vi "Text control 1 v0.1.vi"() -> ()   [LabVIEW 2016]
panel:
  in  "Panel Controls 2":T1={"Emergency Stop"=refnum, "TransGraph Max"=1e-05, "Text/Graph (text=false)"=TRUE, "TransGraph Min"=1e-11} {"TransGraph Min" format="%.2e"; "TransGraph Max" format="%.2e"}
  out "Currently running:":string="#output s 0 0 0 -0.008 0.008 0.002"
  in  "Lines left to run:":string
  in  "Standby":T2
  in  "Full Reset":bool
  in  "SMU4":cluster{"on/off":bool, "Voltage":dbl} {"Voltage" min=-100.0 max=100.0 format="%.2f"}
  in  "Source/Drain\nRange":u8(slide)=6 max=11 scale=0.0..11.0
  in  "Source/Drain\nRange mode":u16(ring) items=["Auto", "Limited", "Fixed"]
  in  "Gate Range":u8(slide)=6 max=11 scale=0.0..11.0
  in  "Gate Range\nmode":u16(ring) items=["Auto", "Limited", "Fixed"]
  in  "Gate":T3={"Gate Start"=0.0, "Gate Stop"=2.0, "Gate Step (linear only)"=1.0, "Gate Compliance"=0.0001, "Gate PComp"=0.0, "Range mode"=0, "Range"=6} {"Range" max=11 scale=0.0..11.0; "Range mode" items=["Auto", "Limited", "Fixed"]; "Gate PComp" format="%^.2e"; "Gate Compliance" format="%^.2e"; "Gate Step (linear only)" format="%^.4e"; "Gate Stop" format="%^.4e"; "Gate Start" format="%^.4e"}
  in  "Drain 2":T4={"Drain Start"=0.0, "Drain Stop"=2.0, "Drain Compliance"=0.0001, "Drain Step"=1.0, "Drain PComp"=0.0, "Range mode"=0, "Range"=6} {"Range" max=11 scale=0.0..11.0; "Range mode" items=["Auto", "Limited", "Fixed"]; "Drain PComp" format="%^.2e"; "Drain Step" format="%^.4e"; "Drain Compliance" format="%^.2e"; "Drain Stop" format="%^.4e"; "Drain Start" format="%^.4e"}
  in  "Timings 2":T5={"integration time"=0, "Short/Long integration time"=0.00064, "hold time (sec)"=0.0, "delay time (sec)"=0.0, "Step Time (0 disables)"=0.0, "sweep method"=0, "Pulse period"=0.005, "Base voltage"=0.0, "Pulse width"=0.0005} {"Pulse width" min=0.0005 max=0.1 step=0.0001 format="%.4f"; "Base voltage" format="%^.4e"; "Pulse period" min=0.005 max=1.0 step=0.0001 format="%.4f"; "sweep method" items=["Continuous", "Pulsed"]; "Step Time (0 disables)" format="%.2f"; "delay time (sec)" format="%.4f"; "hold time (sec)" format="%.4f"; "Short/Long integration time" format="%^.0e"; "integration time" scale=0.0..2.0}
  in  "Panel Controls":T6={"Emergency Stop"=refnum, "TransGraph Max"=1e-05, "Text/Graph (text=false)"=TRUE} {"TransGraph Max" format="%.2e"}
  in  "Interrupt run":bool
  in  "Drain: Compliance":dbl=0.001 format="%.8f"
  in  "Gate: Compliance":dbl=0.001 format="%.8f"
  out "Path":path=path "C:/users/rlp38/09Apr2009LTtesting/test2.txt"
  in  "hold time /s":dbl format="%.2f"
  in  "delay time /s":dbl format="%.2f"
  in  "integration time":u32(slide)=1 max=2 step=1 scale=0.0..2.0
  in  "Integration time (short)":dbl=0.0019 min=8e-05 max=0.0019 step=8e-05 format="%^.0e"
  in  "Integration time (long)":dbl=0.32 min=0.04 max=2.0 step=0.02 format="%.2f"
  in  "Step delay /s":dbl format="%.2f"
  in  "Program":string="#pulsedstressV d 0.03 20 0 0.5 0.0827 5\n#\n#itime m\n#gaterangemode a\n#drainrangemode a\n#pulsed on 0.05 0 0.02\n#transfer d -10 40 1 5 40 35\n#transfer d -10 40 1 5 40 35\n#transfer d -10 40 1 5 40 35\n#output d 0 40 20 0 40 1\n#\n#\n#sample 1 0.008 221 6 0.003\n#samplei 400e-6 200 6 0.002 0.1\n#vsu2pulse -10 4\n#\n#stressV 0.016 0.03 2e-4 0.1e-3 11\n#stressI 220e-7 0.08 15\n#transfer s -1 1 0.5 -0.005 0.005 0.005\n#output s 0 0 0 -0.008 0.008 0.002\n"
  # "Syntax:\nitime [s|m|l]\ngaterangemode [a|l|f]\ndrainrangemode [a|l|f]\npulsed [on|off] PulsePeriod(sec) PulseBaseVoltage PulseONWidth(sec)\nstandby [on l off]\nwait NumMilliseconds\nwait-min NumMinutes\n# texthere = comment\ntransfer [s|d] VgStart VgStop VgStep VdStart VdStop VdStep\noutput [s|d] VgStart VgStop VgStep VdStart VdStop VdStep\nsample Vg Vd NumSamples Time(s) SampleInterval(s)\nsamplei Idg NumSamples Time(s) SampleInterval(s) VDGcompliance\n# if in doubt use SampleInterval(s) = 0.004\nstressV VG VD IGcompliance IDcompliance Duration(sec)\nstressI IDG VDGcompliance Duration(sec)\nvsu2pulse Bias Duration(s)\npulsedstressV [s|d] VEstop VgON VgOFF Period(s) PulseONwidth(s) Vd\nsample-fpp Vg Vd NumSamples Time\nresample-fpp Vg Vd\ntransfer-fpp [s|d] VgStart VgStop VgStep VdStart VdStop VdStep\noutput-fpp [s|d] VgStart VgStop VgStep VdStart VdStop VdStep"
  # "100 samples is approx 13s with medium integration"
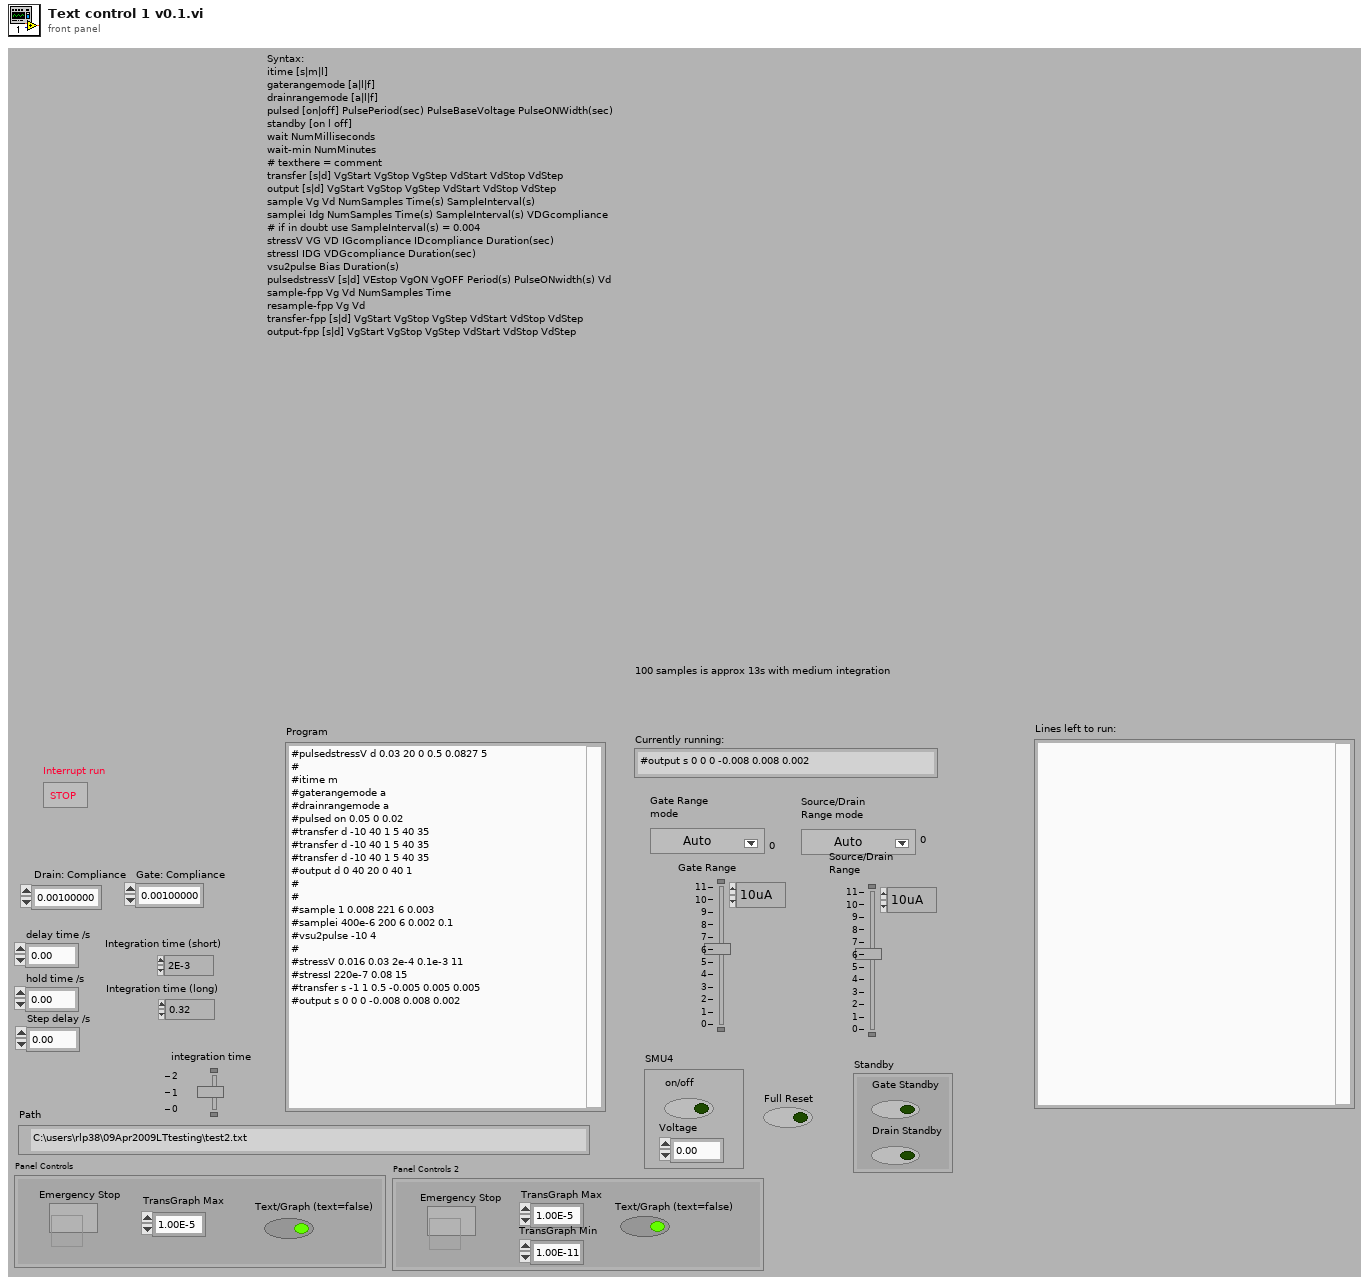
[diagram p1: front panel]
types:
  T1 = cluster{"Emergency Stop":refnum<vi>, "TransGraph Max":dbl, "Text/Graph (text=false)":bool, "TransGraph Min":dbl}
  T2 = cluster{"Gate Standby":bool, "Drain Standby":bool}
  T3 = cluster{"Gate Start":dbl, "Gate Stop":dbl, "Gate Step (linear only)":dbl, "Gate Compliance":dbl, "Gate PComp":dbl, "Range mode":u16, "Range":u8}
  T4 = cluster{"Drain Start":dbl, "Drain Stop":dbl, "Drain Compliance":dbl, "Drain Step":dbl, "Drain PComp":dbl, "Range mode":u16, "Range":u8}
  T5 = cluster{"integration time":u32, "Short/Long integration time":dbl, "hold time (sec)":dbl, "delay time (sec)":dbl, "Step Time (0 disables)":dbl, "sweep method":u16, "Pulse period":dbl, "Base voltage":dbl, "Pulse width":dbl}
  T6 = cluster{"Emergency Stop":refnum<vi>, "TransGraph Max":dbl, "Text/Graph (text=false)":bool}
  T7 = enum16{"open", "replace", "create", "open or create", "replace or create", "replace or create with confirmation"}
  T8 = cluster{"V2 Start":dbl, "V2 Step":dbl, "Number of points":i32}
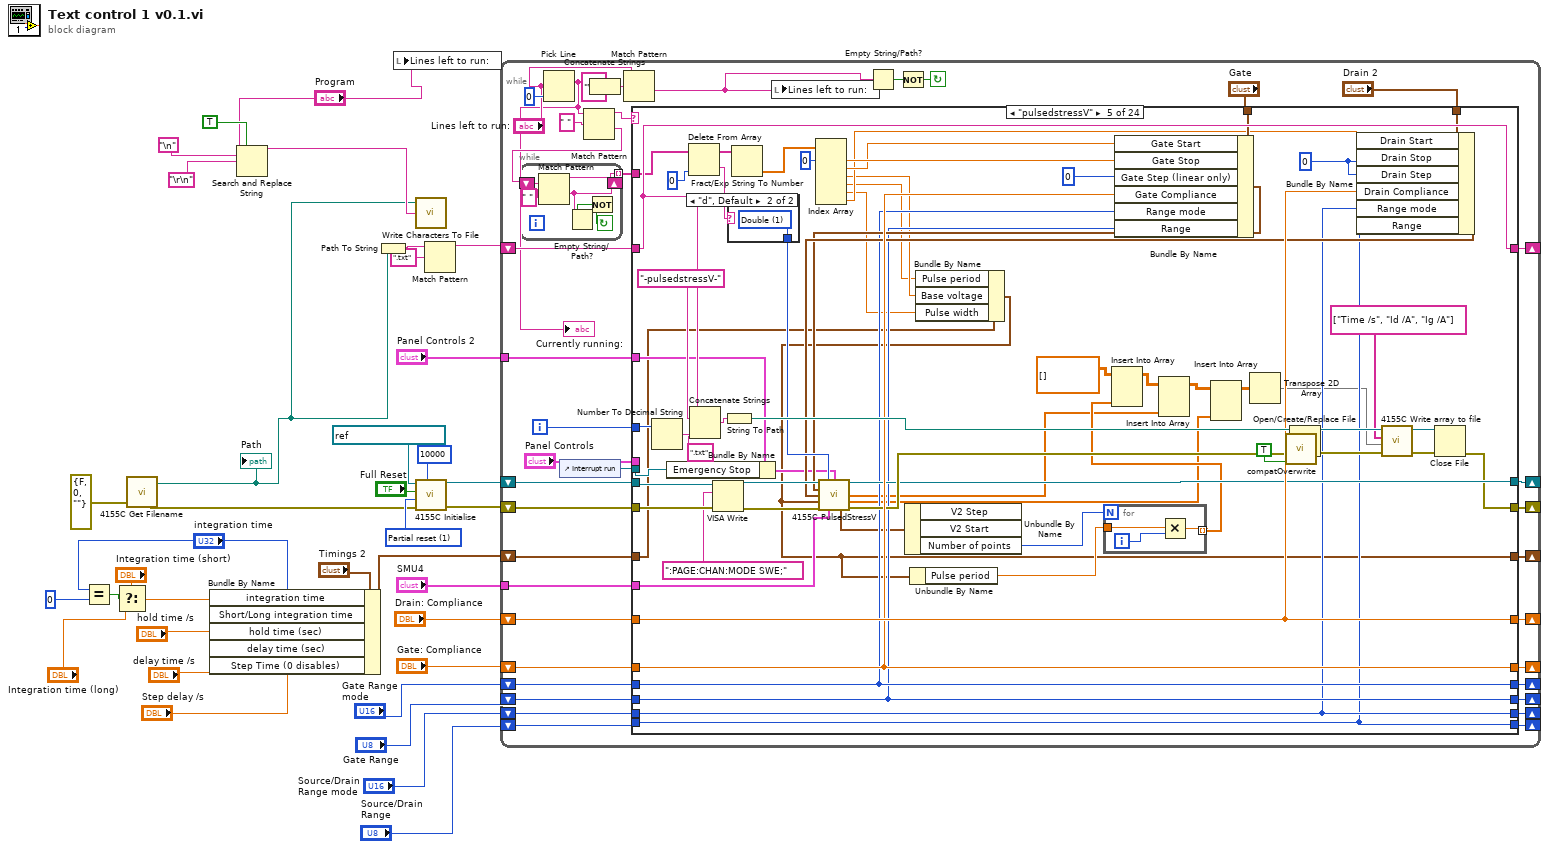
[diagram p0: block diagram]
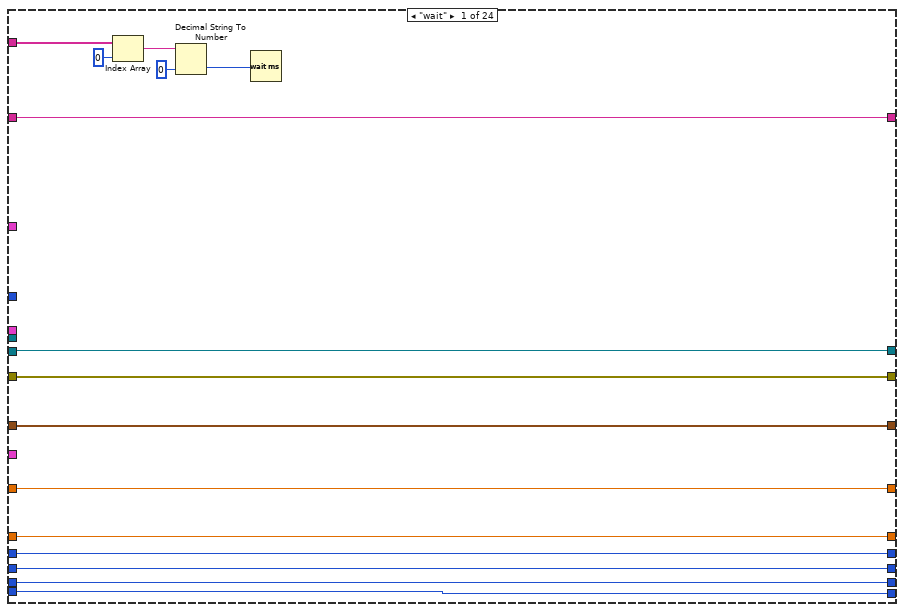
[diagram p2: hidden frame]
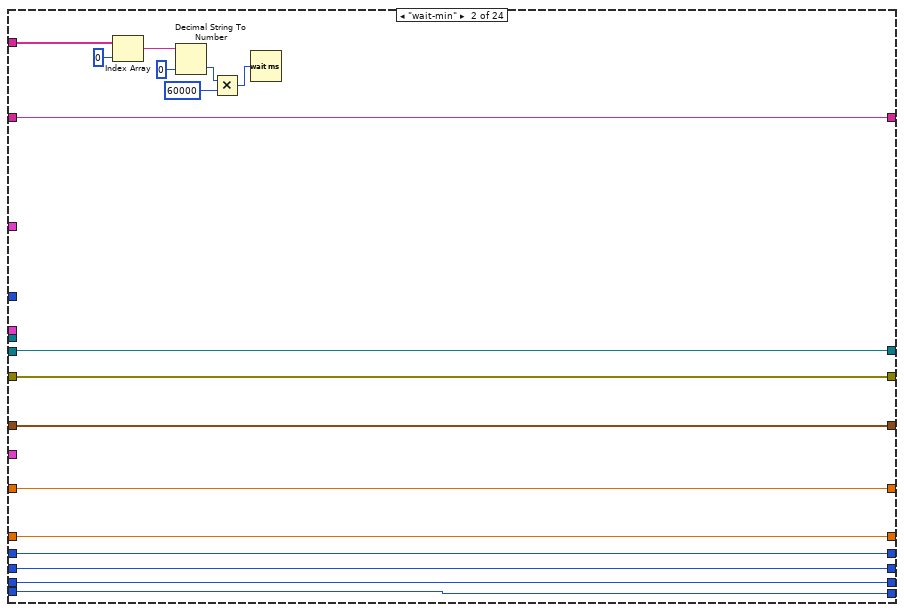
[diagram p3: hidden frame]
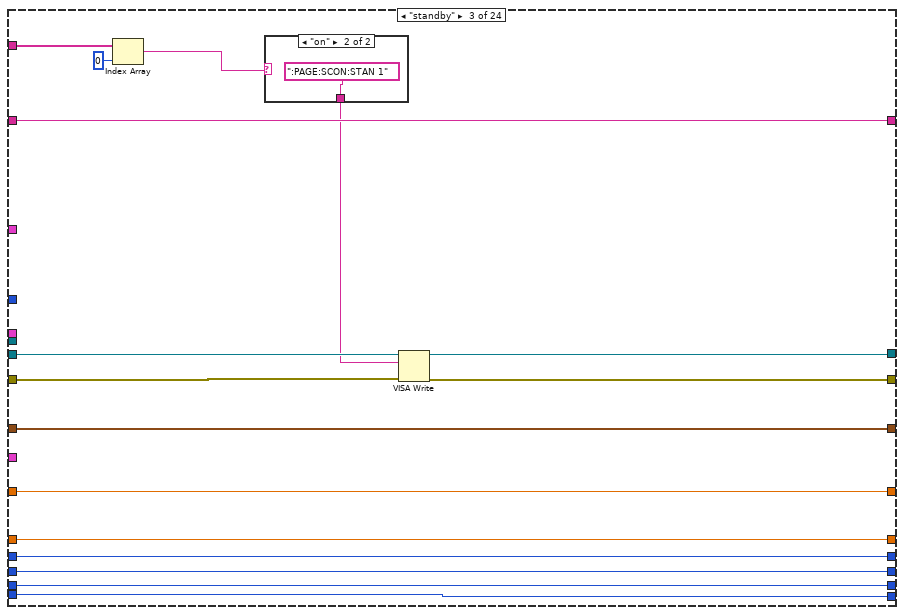
[diagram p4: hidden frame]
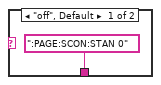
[diagram p5: hidden frame]
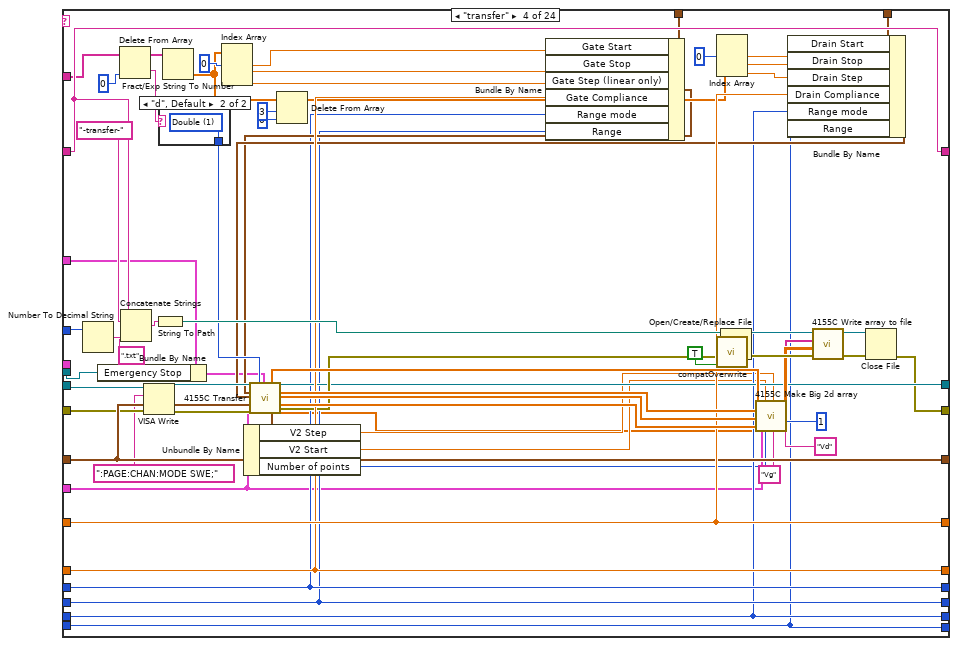
[diagram p6: hidden frame]
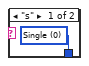
[diagram p7: hidden frame]
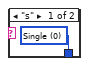
[diagram p8: hidden frame]
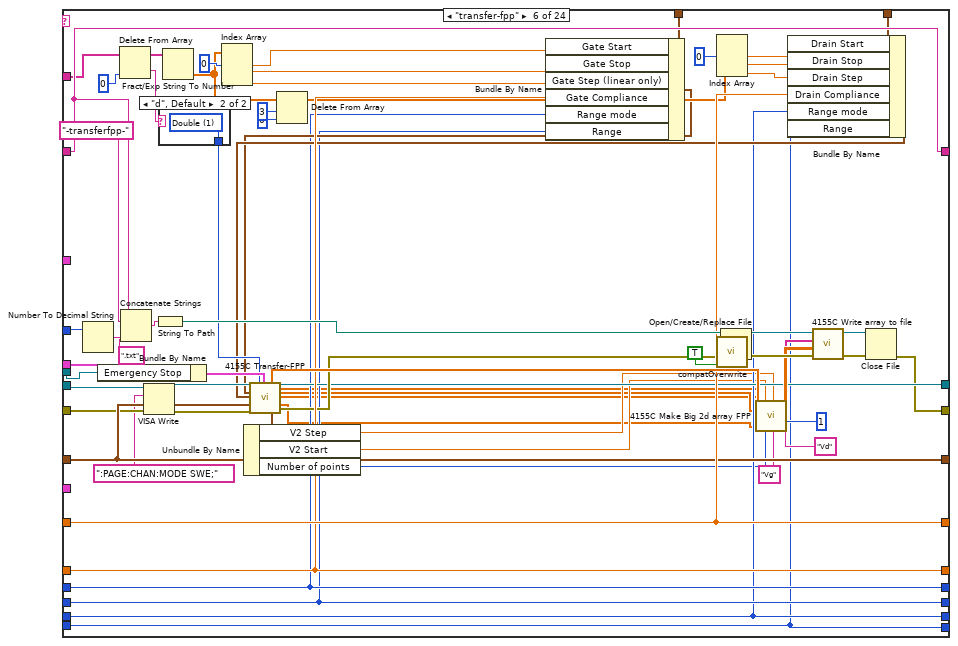
[diagram p9: hidden frame]
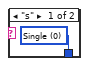
[diagram p10: hidden frame]
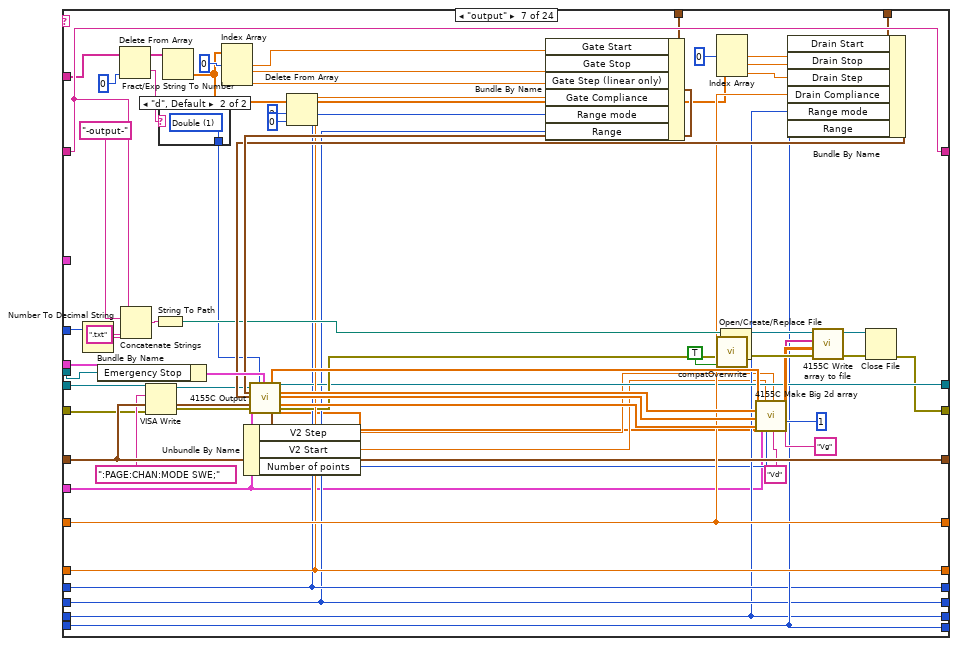
[diagram p11: hidden frame]
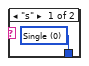
[diagram p12: hidden frame]
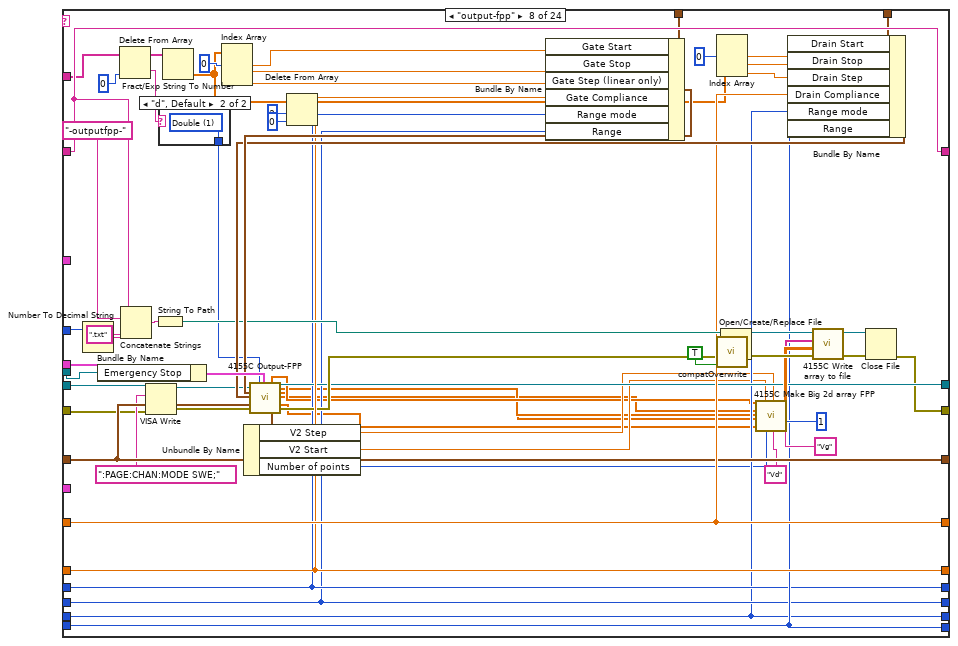
[diagram p13: hidden frame]
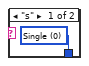
[diagram p14: hidden frame]
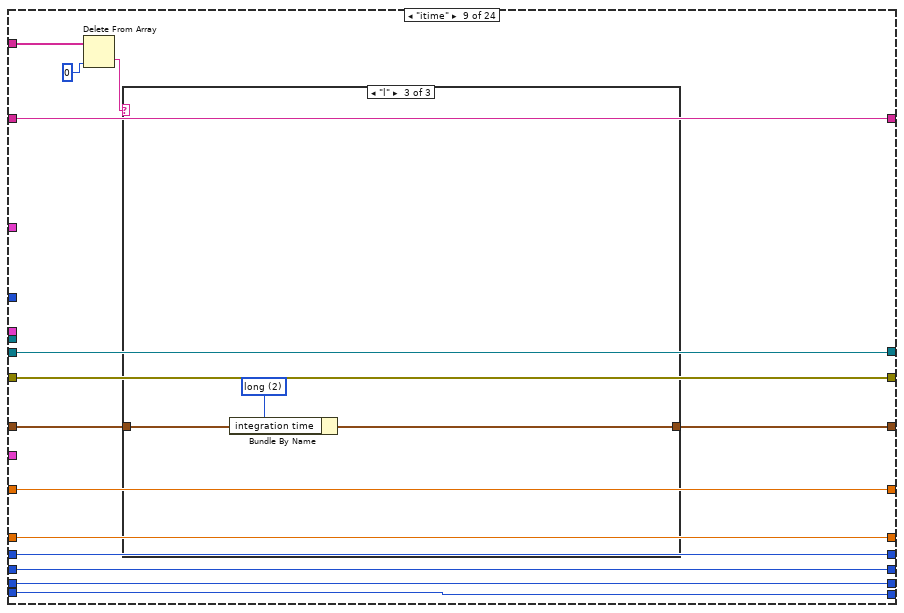
[diagram p15: hidden frame]
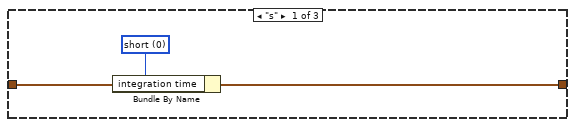
[diagram p16: hidden frame]
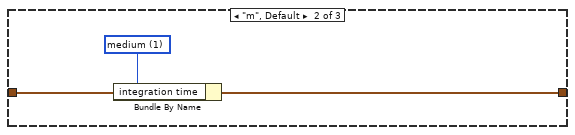
[diagram p17: hidden frame]
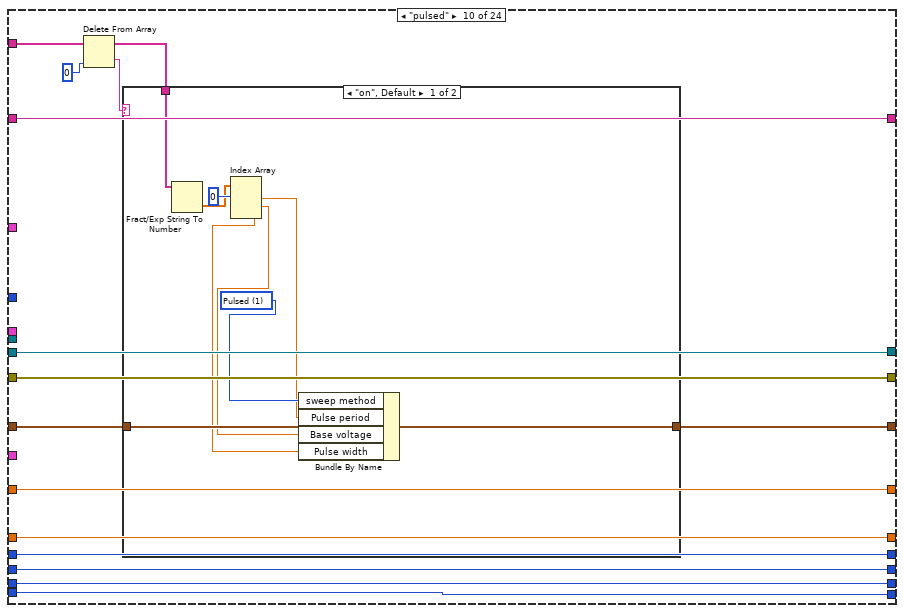
[diagram p18: hidden frame]
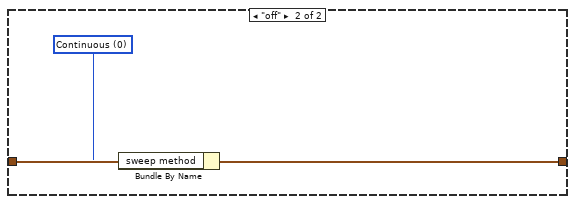
[diagram p19: hidden frame]
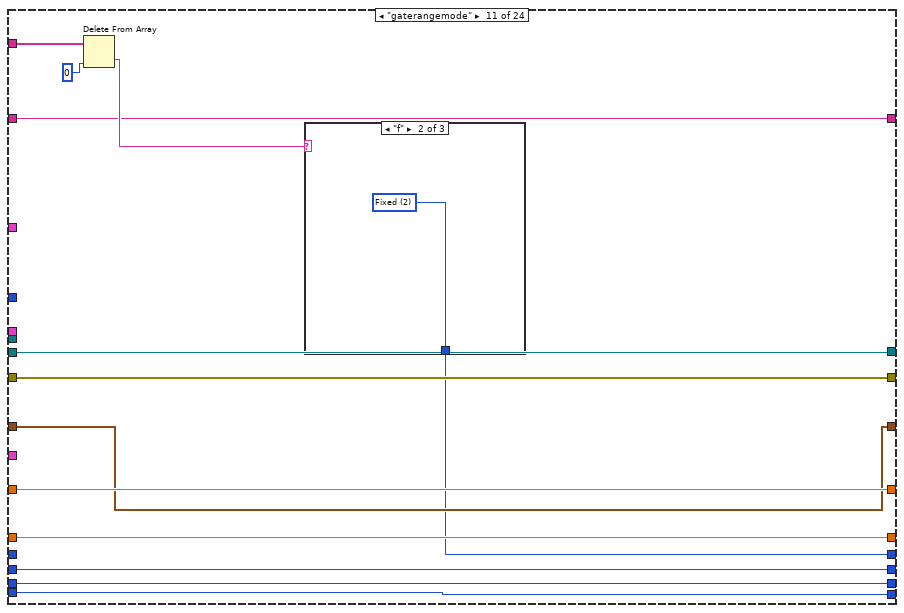
[diagram p20: hidden frame]
diagram:
  w27 = u16 1 items=["Reset All", "Partial reset"] ("Type of reset")
  n1 = Equal?(x="integration time", y=u32 0) -> (x = y?=w31:bool)
  n2 = Select(t="Integration time (short)", s=w31, f="Integration time (long)") -> (s? t:f=w35:dbl)
  n3 = call "4155C Get Filename.vi"("error in (no error)"=errorcluster {"status"=FALSE, "code"=0, "source"=""}) -> ("error out"=w22:errorcluster, "path"=w6:path)  [unwired: 2 in, 1 out]
  "Path" <- w6
  n4 = Bundle By Name(cluster="Timings 2", "integration time"="integration time", "Short/Long integration time"=w35, "hold time (sec)"="hold time /s", "delay time (sec)"="delay time /s", "Step Time (0 disables)"="Step delay /s") -> (w19:T5)
  n5 = Search and Replace String(replace all?=TRUE ("replace all? (F)"), input string="Program", search string="\n", replace string="\r\n") -> (result string=w9:string)  [unwired: 4 in, 3 out]
  n6 = Path To String(path=w6) -> (string=w5:string)
  n7 = local write "Lines left to run:"("Program") -> ()
  n8 = call <vilib>:"Write Characters To File.vi"("character string"=w9, "file path (dialog if empty)"=w6) -> ()  [unwired: 3 in, 1 out]
  n9 = call "4155C Initialise.vi"("VISA resource name in"=refnum<visa-resource-name> "GPIB0::14::INSTR", "Reset"="Full Reset", "Type of reset"=w27, "error in (no error)"=w22, "VISA Timeout Value"=u32 10000) -> ("VISA Resource Name out"=w21:refnum<visa-resource-name>, "error out"=w20:errorcluster)
  n10 = Match Pattern(string=w5, regular expression=".txt") -> (before substring=w4:string)  [unwired: 1 in, 3 out]
  n11 = while {
    tunnel: "SMU4" -> [w41]
    shift-left: "Source/Drain\nRange" -> [w46]
    shift-right: [w42] -> _
    shift-left: "Source/Drain\nRange mode" -> [w47]
    shift-right: [w43] -> _
    shift-left: "Gate Range" -> [w48]
    shift-right: [w44] -> _
    shift-left: "Gate Range\nmode" -> [w49]
    shift-right: [w45] -> _
    shift-left: "Gate: Compliance" -> [w61]
    shift-right: [w55] -> _
    shift-left: "Drain: Compliance" -> [w62]
    shift-right: [w56] -> _
    shift-left: w19 -> [w63]
    shift-right: [w57] -> _
    shift-left: w20 -> [w64]
    shift-right: [w58] -> _
    shift-left: w21 -> [w65]
    shift-right: [w59] -> _
    shift-left: w4 -> [w66]
    shift-right: [w54] -> _
    tunnel: "Panel Controls 2" -> [w37]
    i -> [w60]
    stop <- w74 continue-if-true
    n12 = Pick Line(multi-line string="Lines left to run:", line index=0) -> (output string=w38:string)  [unwired: 1 in]
    "Currently running:" <- w38
    n13 = control-ref of="Interrupt run"() -> (w53:refnum<vi>)
    n14 = Match Pattern(string=w38, regular expression=" ") -> (before substring=w69:string, after substring=w68:string)  [unwired: 1 in, 2 out]
    n15 = while {
      tunnel: [w76] -> w67 mode=indexing
      shift-left: w68 -> [w78]
      shift-right: [w77] -> _
      stop <- w80 continue-if-true
      n16 = Match Pattern(string=w78, regular expression=" ") -> (before substring=w76:string, after substring=w77:string)  [unwired: 1 in, 2 out]
      n17 = Empty String/Path?(string/path=w77) -> (empty?=w81:bool)
      n18 = Not(x=w81) -> (.not. x?=w80:bool)
    }
    n19 = Concatenate Strings(w38, "\n" ("Substring")) -> (w72:string)
    n20 = Match Pattern(string="Lines left to run:", regular expression=w72) -> (after substring=w39:string)  [unwired: 1 in, 3 out]
    n21 = case shown="\"pulsedstressV\"" w69 {
      tunnel: w67 -> [w96 w113 w129 w174 w247 w313 w377 w449 w486 w510 w535 w558 w577 w589 _ _ w684 w742 _ w802 w843 w882 w949 w1008]
      tunnel: w66 -> [w91 w109 w127 w182 w254 w321 w385 w457 w475 w499 w527 w551 w571 w582 w599 w637 w662 w724 w754 w789 w830 w870 w943 w1004]
      tunnel: w65 -> [w90 w108 w118 w152 w238 w290 w353 w425 w476 w500 w528 w552 w572 w583 w604 w640 w691 w749 w758 w809 w850 w889 w956 w961]
      tunnel: w64 -> [w89 w107 w117 w151 w237 w289 w350 w422 w477 w501 w529 w553 w573 w584 w603 w609 w690 w748 w757 w808 w849 w888 w955 w960]
      tunnel: w63 -> [w88 w106 w126 w178 w212 w317 w381 w453 w485 w509 w526 w550 w570 w581 w602 w633 w653 w716 w763 w782 w823 w863 w942 w1003]
      tunnel: w62 -> [w87 w105 w125 w180 w252 w319 w383 w455 w484 w508 w534 w557 w576 w588 w601 w618 w689 w747 w766 w807 w848 w887 w954 w1013]
      tunnel: w61 -> [w86 w104 w124 w179 w251 w318 w382 w454 w483 w507 w533 w556 w575 w587 w600 w619 w663 w725 w765 w790 w831 w871 w944 w1005]
      tunnel: w60 -> [_ _ _ w183 w255 w322 w386 w458 _ _ _ _ _ _ _ w635 w688 w746 _ w806 w847 w886 w953 w1012]
      tunnel: [w90 w108 w116 w176 w249 w315 w379 w451 w476 w500 w528 w552 w572 w583 w604 w640 w654 w697 w756 w783 w824 w864 w894 w963] -> w59
      tunnel: [w89 w107 w115 w175 w248 w314 w378 w450 w477 w501 w529 w553 w573 w584 w603 w608 w664 w698 w755 w791 w832 w872 w893 w962] -> w58
      tunnel: [w88 w106 w126 w178 w208 w317 w381 w453 w478 w502 w526 w550 w570 w581 w602 w633 w653 w716 w763 w782 w823 w863 w942 w1003] -> w57
      tunnel: [w87 w105 w125 w180 w252 w319 w383 w455 w484 w508 w534 w557 w576 w588 w601 w618 w689 w747 w766 w807 w848 w887 w954 w1013] -> w56
      tunnel: [w86 w104 w124 w179 w251 w318 w382 w454 w483 w507 w533 w556 w575 w587 w600 w619 w663 w725 w765 w790 w831 w871 w944 w1005] -> w55
      tunnel: [w91 w109 w127 w182 w254 w321 w385 w457 w475 w499 w527 w551 w571 w582 w599 w637 w662 w724 w754 w789 w830 w870 w943 w1004] -> w54
      tunnel: w53 -> [_ _ _ w191 w259 w327 w394 w462 _ _ _ _ _ _ _ _ w659 w721 _ w788 w829 w869 w914 w979]
      tunnel: "Gate" -> [_ _ _ w161 w241 w300 w364 w436 _ _ _ _ _ _ _ _ _ _ _ _ _ _ _ _]
      tunnel: "Drain 2" -> [_ _ _ w160 w240 w299 w363 w435 _ _ _ _ _ _ _ _ _ _ _ _ _ _ _ _]
      tunnel: "Panel Controls" -> [_ _ _ _ _ w298 w362 w434 _ _ _ _ _ _ _ _ _ _ _ _ _ _ _ _]
      tunnel: w49 -> [w85 w103 w123 w145 w231 w283 w348 w420 w482 w506 _ w549 w569 w580 w598 w620 w649 w712 w759 w778 w819 w859 w938 w999]
      tunnel: w48 -> [w84 w102 w122 w144 w230 w282 w347 w419 w481 w505 w532 _ w560 w586 w597 w621 w650 w713 w760 w779 w820 w860 w939 w1000]
      tunnel: w47 -> [w83 w101 w121 w143 w229 w281 w346 w418 w480 w504 w531 w555 w574 _ w596 w622 w651 w714 w761 w780 w821 w861 w940 w1001]
      tunnel: w46 -> [w82 w100 w120 w142 w228 w280 w349 w421 w479 w503 w530 w554 _ w585 w595 w623 w652 w715 w762 w781 w822 w862 w941 w1002]
      tunnel: [w85 w103 w123 w145 w231 w283 w348 w420 w482 w506 w525 w549 w569 w580 w598 w620 w649 w712 w759 w778 w819 w859 w938 w999] -> w45
      tunnel: [w84 w102 w122 w144 w230 w282 w347 w419 w481 w505 w532 w541 w560 w586 w597 w621 w650 w713 w760 w779 w820 w860 w939 w1000] -> w44
      tunnel: [w83 w101 w121 w143 w229 w281 w346 w418 w480 w504 w531 w555 w574 w579 w596 w622 w651 w714 w761 w780 w821 w861 w940 w1001] -> w43
      tunnel: [w82 w100 w120 w142 w228 w280 w349 w421 w479 w503 w530 w554 w561 w585 w595 w623 w652 w715 w762 w781 w822 w862 w941 w1002] -> w42
      tunnel: w41 -> [_ _ _ w135 w224 _ w340 _ _ _ _ _ _ _ _ _ _ _ _ _ _ _ _ _]
      tunnel: w37 -> [_ _ _ w133 w223 _ _ _ _ _ _ _ _ _ _ _ _ _ _ _ _ _ _ _]
      frame "wait" {
        n22 = Index Array(array=w96, index=0 ("Index")) -> (element=w94:string)
        n23 = Decimal String To Number(string=w94, default (0L)=u32 0) -> (number=w93:u32)  [unwired: 1 in, 1 out]
        n24 = Wait (ms)(milliseconds to wait=w93) -> ()  [unwired: 1 out]
      }
      frame "wait-min" {
        n25 = Index Array(array=w113, index=0 ("Index")) -> (element=w111:string)
        n26 = Decimal String To Number(string=w111, default (0L)=u32 0) -> (number=w99:u32)  [unwired: 1 in, 1 out]
        n27 = Multiply(x=w99, y=u32 60000) -> (x*y=w98:u32)
        n28 = Wait (ms)(milliseconds to wait=w98) -> ()  [unwired: 1 out]
      }
      frame "standby" {
        n29 = Index Array(array=w129, index=0 ("Index")) -> (element=w119:string)
        n30 = case shown="\"on\"" w119 {
          tunnel: [":PAGE:SCON:STAN 0" ":PAGE:SCON:STAN 1"] -> w114
          frame "off", Default {
          }
          frame "on" {
          }
        }
        n31 = VISA Write(VISA resource name=w118, write buffer=w114, error in (no error)=w117) -> (VISA resource name out=w116:refnum<visa-resource-name>, error out=w115:errorcluster)  [unwired: 1 out]
      }
      frame "transfer" {
        n32 = Number To Decimal String(number=w183) -> (decimal integer string=w184:string)  [unwired: 1 in]
        n33 = Bundle By Name(cluster=w133, "Emergency Stop"=w191) -> (w134:T1)
        n34 = Delete From Array(array=w174, index=0 ("Index")) -> (deleted portion=w172:string, array with subset deleted=w171:string[])  [unwired: 1 in]
        n35 = Concatenate Strings(w182, "-transfer-" ("Substring"), w184, ".txt" ("Substring")) -> (w186:string)
        n36 = VISA Write(VISA resource name=w152, write buffer=":PAGE:CHAN:MODE SWE;" ("write buffer (\"\")"), error in (no error)=w151) -> (VISA resource name out=w149:refnum<visa-resource-name>, error out=w150:errorcluster)  [unwired: 1 out]
        n37 = String To Path(string=w186) -> (path=w181:path)
        n38 = case shown="\"d\", Default" w172 {
          tunnel: [w199 w200] -> w170
          frame "s" {
            w199 = u16 0 items=["Single", "Double"] ("sweep mode")
          }
          frame "d", Default {
            w200 = u16 1 items=["Single", "Double"] ("sweep mode")
          }
        }
        n39 = Fract/Exp String To Number(string=w171) -> (number=w156:dbl[])  [unwired: 3 in, 1 out]
        n40 = Index Array(array=w156, index #1=0 ("Index")) -> (element #1=w169:dbl, element #2=w168:dbl, element #3=w167:dbl)  [unwired: 2 in]
        n41 = Delete From Array(array=w156, length=3 ("Length"), index=0 ("Index")) -> (array with subset deleted=w154:dbl[])  [unwired: 1 out]
        n42 = Bundle By Name(cluster=w161, "Gate Start"=w169, "Gate Stop"=w168, "Gate Step (linear only)"=w167, "Gate Compliance"=w179, "Range mode"=w145, "Range"=w144) -> (w146:T3)
        n43 = Index Array(array=w154, index #1=0 ("Index")) -> (element #1=w164:dbl, element #2=w163:dbl, element #3=w162:dbl)  [unwired: 2 in]
        n44 = call <vilib>:"compatOverwrite.vi"("overwrite (F)"=TRUE) -> ("overwrite?"=w132:T7)
        n45 = Bundle By Name(cluster=w160, "Drain Start"=w164, "Drain Stop"=w163, "Drain Step"=w162, "Drain Compliance"=w180, "Range mode"=w143, "Range"=w142) -> (w147:T4)
        n46 = call "4155C Transfer.vi"("VISA resource name in"=w149, "Gate"=w146, "Drain"=w147, "Timings"=w178, "error in (no error)"=w150, "SMU4"=w135, "sweep mode"=w170, "Panel Controls"=w134) -> ("VG"=w187:dbl[], "Outparams"=w140:T8, "VISA Resource Name out"=w176:refnum<visa-resource-name>, "IS"=w190:dbl[], "ID"=w189:dbl[], "IG"=w188:dbl[], "error out"=w177:errorcluster, "SMU4"=w136:dbl[])  [unwired: 12 in]
        n47 = Unbundle By Name(w140) -> ("V2 Step"=w139:dbl, "V2 Start"=w138:dbl, "Number of points"=w137:i32)
        n48 = Open/Create/Replace File(file path (use dialog)=w181, error in=w177, operation (0:open)=w132) -> (refnum out=w196:refnum<file>, error out=w197:errorcluster)  [unwired: 3 in, 1 out]
        n49 = call "4155C Make Big 2d array.vi"("1D Var1"=w187, "1d IS"=w190, "1d ID"=w189, "1d IG"=w188, "1d SMU4"=w136, "SMU4"=w135, "VAR2 START"=w138, "Number of VAR2 steps"=w137, "VAR2 STEP"=w139, "VAR1 Name"="Vg", "Decimal places in header"=i8 1, "VAR2 Name"="Vd") -> ("Header array"=w192:string[], "Data array"=w193:dbl[][])  [unwired: 14 in]
        n50 = call "4155C Write array to file.vi"("Byte Stream File Refnum"=w196, "Header"=w192, "Data Array"=w193, "error in (no error)"=w197) -> ("dup refnum"=w194:refnum<file>, "error out"=w195:errorcluster)  [unwired: 1 in]
        n51 = Close File(refnum=w194, error in=w195) -> (error out=w175:errorcluster)  [unwired: 1 out]
      }
      frame "pulsedstressV" {
        w206 = 0
        n52 = Number To Decimal String(number=w255) -> (decimal integer string=w256:string)  [unwired: 1 in]
        n53 = Bundle By Name(cluster=w223, "Emergency Stop"=w259) -> (w225:T1)
        n54 = Delete From Array(array=w247, index=0 ("Index")) -> (deleted portion=w245:string, array with subset deleted=w244:string[])  [unwired: 1 in]
        n55 = Concatenate Strings(w254, "-pulsedstressV-" ("Substring"), w256, ".txt" ("Substring")) -> (w258:string)
        n56 = VISA Write(VISA resource name=w238, write buffer=":PAGE:CHAN:MODE SWE;" ("write buffer (\"\")"), error in (no error)=w237) -> (VISA resource name out=w235:refnum<visa-resource-name>, error out=w236:errorcluster)  [unwired: 1 out]
        n57 = String To Path(string=w258) -> (path=w253:path)
        n58 = case shown="\"d\", Default" w245 {
          tunnel: [w268 w269] -> w243
          frame "s" {
            w268 = u16 0 items=["Single", "Double"] ("sweep mode")
          }
          frame "d", Default {
            w269 = u16 1 items=["Single", "Double"] ("sweep mode")
          }
        }
        n59 = Fract/Exp String To Number(string=w244) -> (number=w239:dbl[])  [unwired: 3 in, 1 out]
        n60 = Index Array(array=w239, index #1=0 ("Index")) -> (element #1=w215:dbl, element #2=w214:dbl, element #3=w211:dbl, element #4=w210:dbl, element #5=w209:dbl, element #6=w213:dbl)  [unwired: 5 in]
        n61 = Bundle By Name(cluster=w212, "Pulse period"=w210, "Base voltage"=w211, "Pulse width"=w209) -> (w208:T5)
        n62 = Unbundle By Name(w208) -> ("Pulse period"=w216:dbl)
        n63 = Bundle By Name(cluster=w241, "Gate Start"=w214, "Gate Stop"=w215, "Gate Step (linear only)"=0, "Gate Compliance"=w251, "Range mode"=w231, "Range"=w230) -> (w232:T3)
        n64 = call <vilib>:"compatOverwrite.vi"("overwrite (F)"=TRUE) -> ("overwrite?"=w201:T7)
        n65 = Bundle By Name(cluster=w240, "Drain Start"=w213, "Drain Stop"=w206, "Drain Step"=w206, "Drain Compliance"=w252, "Range mode"=w229, "Range"=w228) -> (w233:T4)
        n66 = call "4155C PulsedStressV.vi"("VISA resource name in"=w235, "sweep mode"=w243, "Panel Controls"=w225, "Gate"=w232, "Drain"=w233, "Timings"=w208, "error in (no error)"=w236, "SMU4"=w224) -> ("VISA Resource Name out"=w249:refnum<visa-resource-name>, "ID"=w204:dbl[], "IG"=w202:dbl[], "Outparams"=w226:T8, "error out"=w250:errorcluster)  [unwired: 3 in]
        n67 = Unbundle By Name(w226) -> ("Number of points"=w203:i32)  [unwired: 2 out]
        n68 = for {
          N: w203 -> [_]
          tunnel: [w265] -> w205 mode=indexing
          tunnel: w216 -> [w267]
          i -> [w266]
          n69 = Multiply(x=w267, y=w266) -> (x*y=w265:dbl)
        }
        n70 = Insert Into Array(array=dbl[][] [] ("Input Array"), new element=w205) -> (w217:dbl[][])  [unwired: 2 in]
        n71 = Insert Into Array(array=w217, new element=w204) -> (w222:dbl[][])  [unwired: 2 in]
        n72 = Insert Into Array(array=w222, new element=w202) -> (w221:dbl[][])  [unwired: 2 in]
        n73 = Transpose 2D Array(2D array=w221) -> (transposed array=w220:dbl[][])
        n74 = Open/Create/Replace File(file path (use dialog)=w253, error in=w250, operation (0:open)=w201) -> (refnum out=w262:refnum<file>, error out=w263:errorcluster)  [unwired: 3 in, 1 out]
        n75 = call "4155C Write array to file.vi"("Byte Stream File Refnum"=w262, "Header"=string[] ["Time /s", "Id /A", "Ig /A"], "Data Array"=w220, "error in (no error)"=w263) -> ("dup refnum"=w260:refnum<file>, "error out"=w261:errorcluster)  [unwired: 1 in]
        n76 = Close File(refnum=w260, error in=w261) -> (error out=w248:errorcluster)  [unwired: 1 out]
      }
      frame "transfer-fpp" {
        n77 = Number To Decimal String(number=w322) -> (decimal integer string=w323:string)  [unwired: 1 in]
        n78 = Bundle By Name(cluster=w298, "Emergency Stop"=w327) -> (w335:T6)
        n79 = Delete From Array(array=w313, index=0 ("Index")) -> (deleted portion=w311:string, array with subset deleted=w310:string[])  [unwired: 1 in]
        n80 = Concatenate Strings(w321, "-transferfpp-" ("Substring"), w323, ".txt" ("Substring")) -> (w325:string)
        n81 = VISA Write(VISA resource name=w290, write buffer=":PAGE:CHAN:MODE SWE;" ("write buffer (\"\")"), error in (no error)=w289) -> (VISA resource name out=w287:refnum<visa-resource-name>, error out=w288:errorcluster)  [unwired: 1 out]
        n82 = String To Path(string=w325) -> (path=w320:path)
        n83 = case shown="\"d\", Default" w311 {
          tunnel: [w336 w337] -> w309
          frame "s" {
            w336 = u16 0 items=["Single", "Double"] ("sweep mode")
          }
          frame "d", Default {
            w337 = u16 1 items=["Single", "Double"] ("sweep mode")
          }
        }
        n84 = Fract/Exp String To Number(string=w310) -> (number=w294:dbl[])  [unwired: 3 in, 1 out]
        n85 = Index Array(array=w294, index #1=0 ("Index")) -> (element #1=w308:dbl, element #2=w307:dbl, element #3=w306:dbl)  [unwired: 2 in]
        n86 = Delete From Array(array=w294, length=3 ("Length"), index=0 ("Index")) -> (array with subset deleted=w292:dbl[])  [unwired: 1 out]
        n87 = Bundle By Name(cluster=w300, "Gate Start"=w308, "Gate Stop"=w307, "Gate Step (linear only)"=w306, "Gate Compliance"=w318, "Range mode"=w283, "Range"=w282) -> (w284:T3)
        n88 = Index Array(array=w292, index #1=0 ("Index")) -> (element #1=w303:dbl, element #2=w302:dbl, element #3=w301:dbl)  [unwired: 2 in]
        n89 = call <vilib>:"compatOverwrite.vi"("overwrite (F)"=TRUE) -> ("overwrite?"=w270:T7)
        n90 = Bundle By Name(cluster=w299, "Drain Start"=w303, "Drain Stop"=w302, "Drain Step"=w301, "Drain Compliance"=w319, "Range mode"=w281, "Range"=w280) -> (w285:T4)
        n91 = call "4155C Transfer-FPP.vi"("VISA resource name in"=w287, "Gate"=w284, "Drain"=w285, "Timings"=w317, "error in (no error)"=w288, "sweep mode"=w309, "Panel Controls"=w335) -> ("VG"=w326:dbl[], "Outparams"=w278:T8, "VISA Resource Name out"=w315:refnum<visa-resource-name>, "Vprobe2"=w274:dbl[], "ID"=w273:dbl[], "IG"=w272:dbl[], "Vprobe1"=w271:dbl[], "error out"=w316:errorcluster)  [unwired: 13 in]
        n92 = Unbundle By Name(w278) -> ("V2 Step"=w277:dbl, "V2 Start"=w276:dbl, "Number of points"=w275:i32)
        n93 = Open/Create/Replace File(file path (use dialog)=w320, error in=w316, operation (0:open)=w270) -> (refnum out=w332:refnum<file>, error out=w333:errorcluster)  [unwired: 3 in, 1 out]
        n94 = call "4155C Make Big 2d array FPP.vi"("1D Var1"=w326, "1d ID"=w273, "1d Vp2"=w274, "1d IG"=w272, "1d Vp1"=w271, "VAR2 START"=w276, "Number of VAR2 steps"=w275, "VAR2 STEP"=w277, "VAR1 Name"="Vg", "Decimal places in header"=i8 1, "VAR2 Name"="Vd") -> ("Header array"=w328:string[], "Data array"=w329:dbl[][])  [unwired: 15 in]
        n95 = call "4155C Write array to file.vi"("Byte Stream File Refnum"=w332, "Header"=w328, "Data Array"=w329, "error in (no error)"=w333) -> ("dup refnum"=w330:refnum<file>, "error out"=w331:errorcluster)  [unwired: 1 in]
        n96 = Close File(refnum=w330, error in=w331) -> (error out=w314:errorcluster)  [unwired: 1 out]
      }
      frame "output" {
        n97 = Number To Decimal String(number=w386) -> (decimal integer string=w387:string)  [unwired: 1 in]
        n98 = Bundle By Name(cluster=w362, "Emergency Stop"=w394) -> (w404:T6)
        n99 = Delete From Array(array=w377, index=0 ("Index")) -> (deleted portion=w375:string, array with subset deleted=w374:string[])  [unwired: 1 in]
        n100 = Concatenate Strings(w385, "-output-" ("Substring"), w387, ".txt" ("Substring")) -> (w389:string)
        n101 = VISA Write(VISA resource name=w353, write buffer=":PAGE:CHAN:MODE SWE;" ("write buffer (\"\")"), error in (no error)=w350) -> (VISA resource name out=w352:refnum<visa-resource-name>, error out=w351:errorcluster)  [unwired: 1 out]
        n102 = String To Path(string=w389) -> (path=w384:path)
        n103 = case shown="\"d\", Default" w375 {
          tunnel: [w405 w406] -> w373
          frame "s" {
            w405 = u16 0 items=["Single", "Double"] ("sweep mode")
          }
          frame "d", Default {
            w406 = u16 1 items=["Single", "Double"] ("sweep mode")
          }
        }
        n104 = Fract/Exp String To Number(string=w374) -> (number=w356:dbl[])  [unwired: 3 in, 1 out]
        n105 = Index Array(array=w356, index #1=0 ("Index")) -> (element #1=w372:dbl, element #2=w371:dbl, element #3=w370:dbl)  [unwired: 2 in]
        n106 = Delete From Array(array=w356, length=3 ("Length"), index=0 ("Index")) -> (array with subset deleted=w355:dbl[])  [unwired: 1 out]
        n107 = Bundle By Name(cluster=w364, "Gate Start"=w372, "Gate Stop"=w371, "Gate Step (linear only)"=w370, "Gate Compliance"=w382, "Range mode"=w348, "Range"=w347) -> (w403:T3)
        n108 = Index Array(array=w355, index #1=0 ("Index")) -> (element #1=w367:dbl, element #2=w366:dbl, element #3=w365:dbl)  [unwired: 2 in]
        n109 = call <vilib>:"compatOverwrite.vi"("overwrite (F)"=TRUE) -> ("overwrite?"=w338:T7)
        n110 = Bundle By Name(cluster=w363, "Drain Start"=w367, "Drain Stop"=w366, "Drain Step"=w365, "Drain Compliance"=w383, "Range mode"=w346, "Range"=w349) -> (w402:T4)
        n111 = call "4155C Output.vi"("VISA resource name in"=w352, "Gate"=w403, "Drain"=w402, "Timings"=w381, "error in (no error)"=w351, "SMU4"=w340, "sweep mode"=w373, "Panel controls"=w404) -> ("VD"=w390:dbl[], "Outparams"=w343:T8, "VISA Resource Name out"=w379:refnum<visa-resource-name>, "IS"=w393:dbl[], "ID"=w392:dbl[], "IG"=w391:dbl[], "error out"=w380:errorcluster, "SMU4"=w339:dbl[])  [unwired: 12 in]
        n112 = Unbundle By Name(w343) -> ("V2 Step"=w344:dbl, "V2 Start"=w342:dbl, "Number of points"=w341:i32)
        n113 = Open/Create/Replace File(file path (use dialog)=w384, error in=w380, operation (0:open)=w338) -> (refnum out=w399:refnum<file>, error out=w400:errorcluster)  [unwired: 3 in, 1 out]
        n114 = call "4155C Make Big 2d array.vi"("1D Var1"=w390, "1d IS"=w393, "1d ID"=w392, "1d IG"=w391, "1d SMU4"=w339, "SMU4"=w340, "VAR2 START"=w342, "Number of VAR2 steps"=w341, "VAR2 STEP"=w344, "VAR1 Name"="Vd", "Decimal places in header"=i8 1, "VAR2 Name"="Vg") -> ("Header array"=w395:string[], "Data array"=w396:dbl[][])  [unwired: 14 in]
        n115 = call "4155C Write array to file.vi"("Byte Stream File Refnum"=w399, "Header"=w395, "Data Array"=w396, "error in (no error)"=w400) -> ("dup refnum"=w397:refnum<file>, "error out"=w398:errorcluster)  [unwired: 1 in]
        n116 = Close File(refnum=w397, error in=w398) -> (error out=w378:errorcluster)  [unwired: 1 out]
      }
      frame "output-fpp" {
        n117 = Number To Decimal String(number=w458) -> (decimal integer string=w459:string)  [unwired: 1 in]
        n118 = Bundle By Name(cluster=w434, "Emergency Stop"=w462) -> (w472:T6)
        n119 = Delete From Array(array=w449, index=0 ("Index")) -> (deleted portion=w447:string, array with subset deleted=w446:string[])  [unwired: 1 in]
        n120 = Concatenate Strings(w457, "-outputfpp-" ("Substring"), w459, ".txt" ("Substring")) -> (w461:string)
        n121 = VISA Write(VISA resource name=w425, write buffer=":PAGE:CHAN:MODE SWE;" ("write buffer (\"\")"), error in (no error)=w422) -> (VISA resource name out=w424:refnum<visa-resource-name>, error out=w423:errorcluster)  [unwired: 1 out]
        n122 = String To Path(string=w461) -> (path=w456:path)
        n123 = case shown="\"d\", Default" w447 {
          tunnel: [w473 w474] -> w445
          frame "s" {
            w473 = u16 0 items=["Single", "Double"] ("sweep mode")
          }
          frame "d", Default {
            w474 = u16 1 items=["Single", "Double"] ("sweep mode")
          }
        }
        n124 = Fract/Exp String To Number(string=w446) -> (number=w428:dbl[])  [unwired: 3 in, 1 out]
        n125 = Index Array(array=w428, index #1=0 ("Index")) -> (element #1=w444:dbl, element #2=w443:dbl, element #3=w442:dbl)  [unwired: 2 in]
        n126 = Delete From Array(array=w428, length=3 ("Length"), index=0 ("Index")) -> (array with subset deleted=w427:dbl[])  [unwired: 1 out]
        n127 = Bundle By Name(cluster=w436, "Gate Start"=w444, "Gate Stop"=w443, "Gate Step (linear only)"=w442, "Gate Compliance"=w454, "Range mode"=w420, "Range"=w419) -> (w471:T3)
        n128 = Index Array(array=w427, index #1=0 ("Index")) -> (element #1=w439:dbl, element #2=w438:dbl, element #3=w437:dbl)  [unwired: 2 in]
        n129 = call <vilib>:"compatOverwrite.vi"("overwrite (F)"=TRUE) -> ("overwrite?"=w407:T7)
        n130 = Bundle By Name(cluster=w435, "Drain Start"=w439, "Drain Stop"=w438, "Drain Step"=w437, "Drain Compliance"=w455, "Range mode"=w418, "Range"=w421) -> (w470:T4)
        n131 = call "4155C Output-FPP.vi"("VISA resource name in"=w424, "Gate"=w471, "Drain"=w470, "Timings"=w453, "error in (no error)"=w423, "sweep mode"=w445, "Panel controls"=w472) -> ("VD"=w412:dbl[], "Outparams"=w415:T8, "VISA Resource Name out"=w451:refnum<visa-resource-name>, "Vprobe2"=w411:dbl[], "ID"=w410:dbl[], "IG"=w409:dbl[], "Vprobe1"=w408:dbl[], "error out"=w452:errorcluster)  [unwired: 13 in]
        n132 = Unbundle By Name(w415) -> ("V2 Step"=w416:dbl, "V2 Start"=w414:dbl, "Number of points"=w413:i32)
        n133 = Open/Create/Replace File(file path (use dialog)=w456, error in=w452, operation (0:open)=w407) -> (refnum out=w467:refnum<file>, error out=w468:errorcluster)  [unwired: 3 in, 1 out]
        n134 = call "4155C Make Big 2d array FPP.vi"("1D Var1"=w412, "1d ID"=w410, "1d Vp2"=w411, "1d IG"=w409, "1d Vp1"=w408, "VAR2 START"=w414, "Number of VAR2 steps"=w413, "VAR2 STEP"=w416, "VAR1 Name"="Vd", "Decimal places in header"=i8 1, "VAR2 Name"="Vg") -> ("Header array"=w463:string[], "Data array"=w464:dbl[][])  [unwired: 15 in]
        n135 = call "4155C Write array to file.vi"("Byte Stream File Refnum"=w467, "Header"=w463, "Data Array"=w464, "error in (no error)"=w468) -> ("dup refnum"=w465:refnum<file>, "error out"=w466:errorcluster)  [unwired: 1 in]
        n136 = Close File(refnum=w465, error in=w466) -> (error out=w450:errorcluster)  [unwired: 1 out]
      }
      frame "itime" {
        n137 = Delete From Array(array=w486, index=0 ("Index")) -> (deleted portion=w487:string)  [unwired: 1 in, 1 out]
        n138 = case shown="\"l\"" w487 {
          tunnel: w485 -> [w491 w493 w496]
          tunnel: [w490 w492 w495] -> w478
          frame "s" {
            w489 = u32 0 items=["short  ", "medium  ", "long  "] ("integration time 2")
            n139 = Bundle By Name(cluster=w491, "integration time"=w489) -> (w490:T5)
          }
          frame "m", Default {
            w494 = u32 1 items=["short  ", "medium  ", "long  "] ("integration time 2")
            n140 = Bundle By Name(cluster=w493, "integration time"=w494) -> (w492:T5)
          }
          frame "l" {
            w497 = u32 2 items=["short  ", "medium  ", "long  "] ("integration time 2")
            n141 = Bundle By Name(cluster=w496, "integration time"=w497) -> (w495:T5)
          }
        }
      }
      frame "pulsed" {
        n142 = Delete From Array(array=w510, index=0 ("Index")) -> (deleted portion=w511:string, array with subset deleted=w498:string[])  [unwired: 1 in]
        n143 = case shown="\"on\", Default" w511 {
          tunnel: w509 -> [w521 w524]
          tunnel: [w520 w523] -> w502
          tunnel: w498 -> [w518 _]
          frame "on", Default {
            w519 = u16 1 items=["Continuous", "Pulsed"] ("sweep method")
            n144 = Fract/Exp String To Number(string=w518) -> (number=w516:dbl[])  [unwired: 3 in, 1 out]
            n145 = Index Array(array=w516, index #1=0 ("Index")) -> (element #1=w515:dbl, element #2=w514:dbl, element #3=w513:dbl)  [unwired: 2 in]
            n146 = Bundle By Name(cluster=w521, "sweep method"=w519, "Pulse period"=w515, "Base voltage"=w514, "Pulse width"=w513) -> (w520:T5)
          }
          frame "off" {
            w522 = u16 0 items=["Continuous", "Pulsed"] ("sweep method")
            n147 = Bundle By Name(cluster=w524, "sweep method"=w522) -> (w523:T5)
          }
        }
      }
      frame "gaterangemode" {
        n148 = Delete From Array(array=w535, index=0 ("Index")) -> (deleted portion=w536:string)  [unwired: 1 in, 1 out]
        n149 = case shown="\"f\"" w536 {
          tunnel: [w538 w539 w540] -> w525
          frame "a", Default {
            w538 = u16 0 items=["Auto", "Limited", "Fixed"] ("Gate Range\nmode 2")
          }
          frame "f" {
            w539 = u16 2 items=["Auto", "Limited", "Fixed"] ("Gate Range\nmode 2")
          }
          frame "l" {
            w540 = u16 1 items=["Auto", "Limited", "Fixed"] ("Gate Range\nmode 2")
          }
        }
      }
      frame "gaterange" {
        (unwired) u8 11 items=["10fA  ", "100fA  ", "1nA  ", "10nA", "100nA", "1uA", "10uA", "100uA", "1mA", "10mA", "100mA", "1A"] ("Gate Range 2")
        n150 = Delete From Array(array=w558, index=0 ("Index")) -> (deleted portion=w548:string)  [unwired: 1 in, 1 out]
        n151 = Scan Value(string=w548, format string="") -> (value=w546:dbl)  [unwired: 1 in, 1 out]
        n152 = Logarithm Base 10(1:w546) -> (0:w545:dbl)
        n153 = Round To Nearest(number=w545) -> (nearest integer value=w544:dbl)
        n154 = Add(x=w544, y=11.0) -> (x+y=w542:dbl)
        n155 = To Unsigned Byte Integer(number=w542) -> (unsigned 8bit integer=w541:u8)
      }
      frame "drainrange" {
        (unwired) u8 11 items=["10fA  ", "100fA  ", "1nA  ", "10nA", "100nA", "1uA", "10uA", "100uA", "1mA", "10mA", "100mA", "1A"] ("Gate Range 2")
        n156 = Delete From Array(array=w577, index=0 ("Index")) -> (deleted portion=w568:string)  [unwired: 1 in, 1 out]
        n157 = Scan Value(string=w568, format string="") -> (value=w566:dbl)  [unwired: 1 in, 1 out]
        n158 = Logarithm Base 10(1:w566) -> (0:w565:dbl)
        n159 = Round To Nearest(number=w565) -> (nearest integer value=w564:dbl)
        n160 = Add(x=w564, y=11.0) -> (x+y=w562:dbl)
        n161 = To Unsigned Byte Integer(number=w562) -> (unsigned 8bit integer=w561:u8)
      }
      frame "drainrangemode" {
        n162 = Delete From Array(array=w589, index=0 ("Index")) -> (deleted portion=w590:string)  [unwired: 1 in, 1 out]
        n163 = case shown="\"f\"" w590 {
          tunnel: [w592 w593 w594] -> w579
          frame "a", Default {
            w592 = u16 0 items=["Auto", "Limited", "Fixed"] ("Gate Range\nmode 2")
          }
          frame "f" {
            w593 = u16 2 items=["Auto", "Limited", "Fixed"] ("Gate Range\nmode 2")
          }
          frame "l" {
            w594 = u16 1 items=["Auto", "Limited", "Fixed"] ("Gate Range\nmode 2")
          }
        }
      }
      frame "Error", Default {
      }
      frame "logfile" {
        n164 = Number To Decimal String(number=w635) -> (decimal integer string=w639:string)  [unwired: 1 in]
        n165 = Concatenate Strings(w637, "logfile" ("Substring"), w639, ".txt" ("Substring")) -> (w634:string)
        n166 = String To Path(string=w634) -> (path=w607:path)
        n167 = Unbundle(w633) -> ("integration time"=w632:u32, "Short/Long integration time"=w631:dbl, "hold time (sec)"=w630:dbl, "delay time (sec)"=w629:dbl, "Step Time (0 disables)"=w628:dbl, "sweep method"=w627:u16, "Pulse period"=w626:dbl, "Base voltage"=w625:dbl, "Pulse width"=w624:dbl)
        n168 = Build Array(w632, w631, w630, w629, w628, w627, w626, w625, w624, w618, w619, w620, w621, w622, w623) -> (w611:dbl[])
        n169 = Insert Into Array(array=dbl[][] [] ("Input Array"), new element=w611) -> (w610:dbl[][])  [unwired: 2 in]
        n170 = call <vilib>:"compatOverwrite.vi"("overwrite (F)"=TRUE) -> ("overwrite?"=w605:T7)
        n171 = Open/Create/Replace File(file path (use dialog)=w607, error in=w609, operation (0:open)=w605) -> (refnum out=w615:refnum<file>, error out=w614:errorcluster)  [unwired: 3 in, 1 out]
        n172 = call "4155C Write array to file.vi"("Byte Stream File Refnum"=w615, "Header"=string[] ["Int Time", "Short/Long Itime", "Hold time", "Delay time", "Step time", "Sweep method", "Pulse period", "Base Voltage", "Pulse width", "Drain compliance", "Gate compliance", "Gate range mode", "Gate range", "S/D range mode", "S/D range"], "Data Array"=w610, "error in (no error)"=w614) -> ("dup refnum"=w617:refnum<file>, "error out"=w616:errorcluster)  [unwired: 1 in]
        n173 = Close File(refnum=w617, error in=w616) -> (error out=w608:errorcluster)  [unwired: 1 out]
      }
      frame "sample" {
        n174 = Number To Decimal String(number=w688) -> (decimal integer string=w687:string)  [unwired: 1 in]
        n175 = Fract/Exp String To Number(string=w684) -> (number=w644:dbl[])  [unwired: 3 in, 1 out]
        n176 = Concatenate Strings(w662, "-sample-" ("Substring"), w687, ".txt" ("Substring")) -> (w685:string)
        n177 = String To Path(string=w685) -> (path=w666:path)
        n178 = Index Array(array=w644, index=0 ("Index")) -> (element=w682:dbl)
        n179 = Index Array(array=w644, index=2 ("Index")) -> (element=w678:dbl)
        n180 = Index Array(array=w644, index=3 ("Index")) -> (element=w647:dbl)
        n181 = Index Array(array=w644, index=4 ("Index")) -> (element=w643:dbl)
        n182 = call "4155C Config Sampling Measurements.vi"("Sampling interval"=w643, "Sample time"=w647, "Display on/off"=TRUE, "Timings"=w653, "Num Points"=w678, "error in (no error)"=w690, "Drain Compliance"=w689, "Gate Compliance"=w663, "VISA session"=w691) -> ("error out"=w692:errorcluster, "dup VISA resource name"=w693:refnum<visa-resource-name>)  [unwired: 1 in]
        n183 = Index Array(array=w644, index=1 ("Index")) -> (element=w679:dbl)
        n184 = call "4155C Take Sample.vi"("Emergency Stop"=w659, "error in (no error)"=w692, "Vd"=w679, "Vg"=w682, "VISA resource name in"=w693) -> ("error out"=w657:errorcluster, "Id"=w695:dbl[], "Ig"=w668:dbl[], "VISA Resource Name out"=w655:refnum<visa-resource-name>, "Is"=w694:dbl[], "Time"=w672:dbl[])  [unwired: 1 in]
        n185 = Insert Into Array(array=dbl[][] [] ("Input Array"), new element=w672) -> (w671:dbl[][])  [unwired: 2 in]
        n186 = Insert Into Array(array=w671, new element=w668) -> (w670:dbl[][])  [unwired: 2 in]
        n187 = Insert Into Array(array=w670, new element=w695) -> (w669:dbl[][])  [unwired: 2 in]
        n188 = VISA Write(VISA resource name=w655, write buffer=":DISP ON" ("write buffer (\"\")"), error in (no error)=w657) -> (VISA resource name out=w654:refnum<visa-resource-name>, error out=w656:errorcluster)  [unwired: 1 out]
        n189 = Insert Into Array(array=w669, new element=w694) -> (w661:dbl[][])  [unwired: 2 in]
        n190 = Transpose 2D Array(2D array=w661) -> (transposed array=w660:dbl[][])
        n191 = call <vilib>:"compatOverwrite.vi"("overwrite (F)"=TRUE) -> ("overwrite?"=w641:T7)
        n192 = Open/Create/Replace File(file path (use dialog)=w666, error in=w656, operation (0:open)=w641) -> (refnum out=w675:refnum<file>, error out=w674:errorcluster)  [unwired: 3 in, 1 out]
        n193 = call "4155C Write array to file.vi"("Byte Stream File Refnum"=w675, "Header"=string[] ["Time /s", "Ig /A", "Id /A", "Is /A"], "Data Array"=w660, "error in (no error)"=w674) -> ("dup refnum"=w677:refnum<file>, "error out"=w676:errorcluster)  [unwired: 1 in]
        n194 = Close File(refnum=w677, error in=w676) -> (error out=w664:errorcluster)  [unwired: 1 out]
      }
      frame "samplei" {
        n195 = Number To Decimal String(number=w746) -> (decimal integer string=w745:string)  [unwired: 1 in]
        n196 = Fract/Exp String To Number(string=w742) -> (number=w708:dbl[])  [unwired: 3 in, 1 out]
        n197 = Concatenate Strings(w724, "-samplei-" ("Substring"), w745, ".txt" ("Substring")) -> (w743:string)
        n198 = String To Path(string=w743) -> (path=w727:path)
        n199 = Index Array(array=w708, index=4 ("Index")) -> (element=w702:dbl)
        n200 = Index Array(array=w708, index=3 ("Index")) -> (element=w703:dbl)
        n201 = Index Array(array=w708, index=1 ("Index")) -> (element=w705:dbl)
        n202 = Index Array(array=w708, index=0 ("Index")) -> (element=w706:dbl)
        n203 = Index Array(array=w708, index=2 ("Index")) -> (element=w704:dbl)
        n204 = call "4155C Config SamplingI Measurements.vi"("Sample time"=w704, "Display on/off"=TRUE, "Timings"=w716, "Num Points"=w705, "error in (no error)"=w748, "Sampling interval"=w703, "VISA session"=w749) -> ("error out"=w750:errorcluster, "dup VISA resource name"=w751:refnum<visa-resource-name>)  [unwired: 3 in]
        n205 = call "4155C Take SampleI.vi"("Emergency Stop"=w721, "error in (no error)"=w750, "Idg 2"=w706, "Vdg compliance 2"=w702, "VISA resource name in"=w751) -> ("error out"=w719:errorcluster, "Idg"=w753:dbl[], "Vdg"=w729:dbl[], "VISA Resource Name out"=w717:refnum<visa-resource-name>, "Is"=w752:dbl[], "Time"=w733:dbl[])  [unwired: 1 in]
        n206 = Insert Into Array(array=dbl[][] [] ("Input Array"), new element=w733) -> (w732:dbl[][])  [unwired: 2 in]
        n207 = Insert Into Array(array=w732, new element=w729) -> (w731:dbl[][])  [unwired: 2 in]
        n208 = Insert Into Array(array=w731, new element=w753) -> (w730:dbl[][])  [unwired: 2 in]
        n209 = VISA Write(VISA resource name=w717, write buffer=":DISP ON" ("write buffer (\"\")"), error in (no error)=w719) -> (VISA resource name out=w701:refnum<visa-resource-name>, error out=w718:errorcluster)  [unwired: 1 out]
        n210 = Insert Into Array(array=w730, new element=w752) -> (w723:dbl[][])  [unwired: 2 in]
        n211 = Transpose 2D Array(2D array=w723) -> (transposed array=w722:dbl[][])
        n212 = call <vilib>:"compatOverwrite.vi"("overwrite (F)"=TRUE) -> ("overwrite?"=w696:T7)
        n213 = Open/Create/Replace File(file path (use dialog)=w727, error in=w718, operation (0:open)=w696) -> (refnum out=w736:refnum<file>, error out=w735:errorcluster)  [unwired: 3 in, 1 out]
        n214 = call "4155C Write array to file.vi"("Byte Stream File Refnum"=w736, "Header"=string[] ["Time /s", "Vdg /V", "Idg /A", "Is /A"], "Data Array"=w722, "error in (no error)"=w735) -> ("dup refnum"=w738:refnum<file>, "error out"=w737:errorcluster)  [unwired: 1 in]
        n215 = Close File(refnum=w738, error in=w737) -> (error out=w699:errorcluster)  [unwired: 1 out]
        n216 = VISA Write(VISA resource name=w701, write buffer=";:PAGE:SCON:STAN OFF;:PAGE:CHAN:VSU2:DIS;" ("write buffer (\"\")"), error in (no error)=w699) -> (VISA resource name out=w697:refnum<visa-resource-name>, error out=w698:errorcluster)  [unwired: 1 out]
      }
      frame "#" {
        n217 = VISA Write(VISA resource name=w758, write buffer=":DISP ON" ("write buffer (\"\")"), error in (no error)=w757) -> (VISA resource name out=w756:refnum<visa-resource-name>, error out=w755:errorcluster)  [unwired: 1 out]
      }
      frame "stressV" {
        n218 = Number To Decimal String(number=w806) -> (decimal integer string=w805:string)  [unwired: 1 in]
        n219 = Fract/Exp String To Number(string=w802) -> (number=w774:dbl[])  [unwired: 3 in, 1 out]
        n220 = Concatenate Strings(w789, "-stressV-" ("Substring"), w805, ".txt" ("Substring")) -> (w803:string)
        n221 = String To Path(string=w803) -> (path=w793:path)
        n222 = Index Array(array=w774, index=3 ("Index")) -> (element=w771:dbl)
        n223 = Index Array(array=w774, index=1 ("Index")) -> (element=w769:dbl)
        n224 = Index Array(array=w774, index=0 ("Index")) -> (element=w768:dbl)
        n225 = Index Array(array=w774, index=4 ("Index")) -> (element=w773:dbl)
        n226 = Index Array(array=w774, index=2 ("Index")) -> (element=w770:dbl)
        n227 = call "4155C Config V Stress.vi"("VISA session"=w809, "ID compliance"=w771, "VD"=w769, "VG"=w768, "IG compliance"=w770, "error in (no error)"=w808, "Display on/off"=TRUE) -> ("dup VISA resource name"=w811:refnum<visa-resource-name>, "error out"=w810:errorcluster)
        n228 = call "4155C Apply Stress.vi"("error in (no error)"=w810, "Duration"=w773, "Emergency Stop"=w788, "VISA resource name in"=w811) -> ("error out"=w786:errorcluster, "VISA Resource Name out"=w784:refnum<visa-resource-name>)
        n229 = VISA Write(VISA resource name=w784, write buffer=":DISP ON" ("write buffer (\"\")"), error in (no error)=w786) -> (VISA resource name out=w783:refnum<visa-resource-name>, error out=w785:errorcluster)  [unwired: 1 out]
        n230 = call <vilib>:"compatOverwrite.vi"("overwrite (F)"=TRUE) -> ("overwrite?"=w767:T7)
        n231 = Open/Create/Replace File(file path (use dialog)=w793, error in=w785, operation (0:open)=w767) -> (refnum out=w796:refnum<file>, error out=w795:errorcluster)  [unwired: 3 in, 1 out]
        n232 = call "4155C Write array to file.vi"("Byte Stream File Refnum"=w796, "Header"=string[] ["V stress completed successfully", ""], "error in (no error)"=w795) -> ("dup refnum"=w798:refnum<file>, "error out"=w797:errorcluster)  [unwired: 2 in]
        n233 = Close File(refnum=w798, error in=w797) -> (error out=w791:errorcluster)  [unwired: 1 out]
      }
      frame "stressI" {
        n234 = Number To Decimal String(number=w847) -> (decimal integer string=w846:string)  [unwired: 1 in]
        n235 = Fract/Exp String To Number(string=w843) -> (number=w817:dbl[])  [unwired: 3 in, 1 out]
        n236 = Concatenate Strings(w830, "-stressI-" ("Substring"), w846, ".txt" ("Substring")) -> (w844:string)
        n237 = String To Path(string=w844) -> (path=w834:path)
        n238 = Index Array(array=w817, index=1 ("Index")) -> (element=w813:dbl)
        n239 = Index Array(array=w817, index=0 ("Index")) -> (element=w814:dbl)
        n240 = call "4155C Config I Stress.vi"("VISA session"=w850, "IDG"=w814, "VDG compliance"=w813, "error in (no error)"=w849, "Display on/off"=TRUE) -> ("dup VISA resource name"=w852:refnum<visa-resource-name>, "error out"=w851:errorcluster)
        n241 = Index Array(array=w817, index=2 ("Index")) -> (element=w815:dbl)
        n242 = call "4155C Apply Stress.vi"("error in (no error)"=w851, "Duration"=w815, "Emergency Stop"=w829, "VISA resource name in"=w852) -> ("error out"=w827:errorcluster, "VISA Resource Name out"=w825:refnum<visa-resource-name>)
        n243 = VISA Write(VISA resource name=w825, write buffer=":DISP ON" ("write buffer (\"\")"), error in (no error)=w827) -> (VISA resource name out=w824:refnum<visa-resource-name>, error out=w826:errorcluster)  [unwired: 1 out]
        n244 = call <vilib>:"compatOverwrite.vi"("overwrite (F)"=TRUE) -> ("overwrite?"=w812:T7)
        n245 = Open/Create/Replace File(file path (use dialog)=w834, error in=w826, operation (0:open)=w812) -> (refnum out=w837:refnum<file>, error out=w836:errorcluster)  [unwired: 3 in, 1 out]
        n246 = call "4155C Write array to file.vi"("Byte Stream File Refnum"=w837, "Header"=string[] ["I stress completed successfully", ""], "error in (no error)"=w836) -> ("dup refnum"=w839:refnum<file>, "error out"=w838:errorcluster)  [unwired: 2 in]
        n247 = Close File(refnum=w839, error in=w838) -> (error out=w832:errorcluster)  [unwired: 1 out]
      }
      frame "vsu2pulse" {
        n248 = Number To Decimal String(number=w886) -> (decimal integer string=w885:string)  [unwired: 1 in]
        n249 = Fract/Exp String To Number(string=w882) -> (number=w857:dbl[])  [unwired: 3 in, 1 out]
        n250 = Concatenate Strings(w870, "-vsu2-" ("Substring"), w885, ".txt" ("Substring")) -> (w883:string)
        n251 = String To Path(string=w883) -> (path=w874:path)
        n252 = Index Array(array=w857, index=1 ("Index")) -> (element=w856:dbl)
        n253 = Index Array(array=w857, index=0 ("Index")) -> (element=w854:dbl)
        n254 = call "4155C Config VSU2 Stress.vi"("error in (no error)"=w888, "VSU2"=w854, "Display on/off"=TRUE, "VISA session"=w889) -> ("error out"=w890:errorcluster, "dup VISA resource name"=w891:refnum<visa-resource-name>)
        n255 = call "4155C Apply Stress.vi"("error in (no error)"=w890, "Duration"=w856, "Emergency Stop"=w869, "VISA resource name in"=w891) -> ("error out"=w867:errorcluster, "VISA Resource Name out"=w865:refnum<visa-resource-name>)
        n256 = VISA Write(VISA resource name=w865, write buffer=":DISP ON" ("write buffer (\"\")"), error in (no error)=w867) -> (VISA resource name out=w864:refnum<visa-resource-name>, error out=w866:errorcluster)  [unwired: 1 out]
        n257 = call <vilib>:"compatOverwrite.vi"("overwrite (F)"=TRUE) -> ("overwrite?"=w853:T7)
        n258 = Open/Create/Replace File(file path (use dialog)=w874, error in=w866, operation (0:open)=w853) -> (refnum out=w877:refnum<file>, error out=w876:errorcluster)  [unwired: 3 in, 1 out]
        n259 = call "4155C Write array to file.vi"("Byte Stream File Refnum"=w877, "Header"=string[] ["VSU2 pulse completed successfully", ""], "error in (no error)"=w876) -> ("dup refnum"=w879:refnum<file>, "error out"=w878:errorcluster)  [unwired: 2 in]
        n260 = Close File(refnum=w879, error in=w878) -> (error out=w872:errorcluster)  [unwired: 1 out]
      }
      frame "sample-fpp" {
        w899 = string[] ["Time /s", "Id VgVd /A", "Ig VgVd /A", "Vp1 VgVd /V", "Vp2 VgVd /V"] ("Header")
        w903 = "%d" ("format string")
        n261 = Number To Decimal String(number=w953) -> (decimal integer string=w952:string)  [unwired: 1 in]
        n262 = Fract/Exp String To Number(string=w949) -> (number=w937:dbl[])  [unwired: 3 in, 1 out]
        n263 = Concatenate Strings(w943, "-samplefpp-" ("Substring"), w952, ".txt" ("Substring")) -> (w950:string)
        n264 = String To Path(string=w950) -> (path=w911:path)
        n265 = Index Array(array=w937, index=0 ("Index")) -> (element=w897:dbl)
        n266 = Index Array(array=w937, index=1 ("Index")) -> (element=w896:dbl)
        n267 = Index Array(array=w937, index=2 ("Index")) -> (element=w945:dbl)
        n268 = Index Array(array=w937, index=3 ("Index")) -> (element=w935:dbl)
        n269 = call "4155C Config Sampling Measurements FPP.vi"("VISA session"=w956, "Num Points"=w945, "Vg"=w897, "Display on/off"=TRUE, "Gate Compliance"=w944, "Drain Compliance"=w954, "Standby"="Standby", "error in (no error)"=w955, "Timings"=w942, "Vd"=w896, "Sample time"=w935) -> ("dup VISA resource name"=w913:refnum<visa-resource-name>, "error out"=w912:errorcluster)  [unwired: 3 in]
        n270 = Number To Decimal String(number=w897) -> (decimal integer string=w923:string)  [unwired: 1 in]
        n271 = call "4155C Take Sample FPP.vi"("VISA resource name in"=w913, "error in (no error)"=w912, "Emergency Stop"=w914) -> ("Time"=w918:dbl[], "Vp1"=w928:dbl[], "VISA Resource Name out"=w894:refnum<visa-resource-name>, "Ig"=w916:dbl[], "Id"=w917:dbl[], "Vp2"=w926:dbl[], "error out"=w915:errorcluster)  [unwired: 10 in]
        n272 = Insert Into Array(array=dbl[][] [] ("Input Array"), new element=w918) -> (w932:dbl[][])  [unwired: 2 in]
        n273 = Number To Decimal String(number=w896) -> (decimal integer string=w921:string)  [unwired: 1 in]
        n274 = Insert Into Array(array=w932, new element=w917) -> (w931:dbl[][])  [unwired: 2 in]
        n275 = Concatenate Strings("(Vg = " ("Substring"), w923, "V, Vd = " ("Substring"), w921, "V)" ("Substring")) -> (w919:string)
        n276 = Insert Into Array(array=w931, new element=w916) -> (w930:dbl[][])  [unwired: 2 in]
        n277 = Insert Into Array(array=w930, new element=w928) -> (w927:dbl[][])  [unwired: 2 in]
        n278 = Insert Into Array(array=w927, new element=w926) -> (w895:dbl[][])  [unwired: 2 in]
        n279 = call <vilib>:"compatOverwrite.vi"("overwrite (F)"=TRUE) -> ("overwrite?"=w892:T7)
        n280 = Open/Create/Replace File(file path (use dialog)=w911, error in=w915, operation (0:open)=w892) -> (refnum out=w908:refnum<file>, error out=w909:errorcluster)  [unwired: 3 in, 1 out]
        n281 = Array To Spreadsheet String(array=w899, 3:w903) -> (spreadsheet string=w905:string)  [unwired: 1 in]
        n282 = Transpose 2D Array(2D array=w895) -> (transposed array=w925:dbl[][])
        n283 = Search and Replace String(replace all?=TRUE ("replace all? (F)"), input string=w905, search string="VgVd", replace string=w919) -> (result string=w901:string)  [unwired: 4 in, 3 out]
        n284 = Spreadsheet String To Array(format string=w903, spreadsheet string=w901, array type (2D Dbl)=w899) -> (array=w900:string[])  [unwired: 1 in]
        n285 = call "4155C Write array to file.vi"("Byte Stream File Refnum"=w908, "Header"=w900, "Data Array"=w925, "error in (no error)"=w909) -> ("dup refnum"=w906:refnum<file>, "error out"=w907:errorcluster)  [unwired: 1 in]
        n286 = Close File(refnum=w906, error in=w907) -> (error out=w893:errorcluster)  [unwired: 1 out]
      }
      frame "resample-fpp" {
        w966 = string[] ["Time /s", "Id VgVd /A", "Ig VgVd /A", "Vp1 VgVd /V", "Vp2 VgVd /V"] ("Header")
        w970 = "%d" ("format string")
        n287 = Number To Decimal String(number=w1012) -> (decimal integer string=w1011:string)  [unwired: 1 in]
        n288 = Fract/Exp String To Number(string=w1008) -> (number=w959:dbl[])  [unwired: 3 in, 1 out]
        n289 = Concatenate Strings(w1004, "-resamplefpp-" ("Substring"), w1011, ".txt" ("Substring")) -> (w1009:string)
        n290 = String To Path(string=w1009) -> (path=w978:path)
        n291 = Index Array(array=w959, index=0 ("Index")) -> (element=w965:dbl)
        n292 = Index Array(array=w959, index=1 ("Index")) -> (element=w964:dbl)
        n293 = Number To Decimal String(number=w965) -> (decimal integer string=w988:string)  [unwired: 1 in]
        n294 = call "4155C Take Sample FPP.vi"("VISA resource name in"=w961, "error in (no error)"=w960, "Emergency Stop"=w979) -> ("Time"=w983:dbl[], "Vp1"=w993:dbl[], "VISA Resource Name out"=w963:refnum<visa-resource-name>, "Ig"=w981:dbl[], "Id"=w982:dbl[], "Vp2"=w991:dbl[], "error out"=w980:errorcluster)  [unwired: 10 in]
        n295 = Insert Into Array(array=dbl[][] [] ("Input Array"), new element=w983) -> (w997:dbl[][])  [unwired: 2 in]
        n296 = Number To Decimal String(number=w964) -> (decimal integer string=w986:string)  [unwired: 1 in]
        n297 = Insert Into Array(array=w997, new element=w982) -> (w996:dbl[][])  [unwired: 2 in]
        n298 = Concatenate Strings("(Vg = " ("Substring"), w988, "V, Vd = " ("Substring"), w986, "V)" ("Substring")) -> (w984:string)
        n299 = Insert Into Array(array=w996, new element=w981) -> (w995:dbl[][])  [unwired: 2 in]
        n300 = Insert Into Array(array=w995, new element=w993) -> (w992:dbl[][])  [unwired: 2 in]
        n301 = Insert Into Array(array=w992, new element=w991) -> (w958:dbl[][])  [unwired: 2 in]
        n302 = call <vilib>:"compatOverwrite.vi"("overwrite (F)"=TRUE) -> ("overwrite?"=w957:T7)
        n303 = Open/Create/Replace File(file path (use dialog)=w978, error in=w980, operation (0:open)=w957) -> (refnum out=w975:refnum<file>, error out=w976:errorcluster)  [unwired: 3 in, 1 out]
        n304 = Array To Spreadsheet String(array=w966, 3:w970) -> (spreadsheet string=w972:string)  [unwired: 1 in]
        n305 = Transpose 2D Array(2D array=w958) -> (transposed array=w990:dbl[][])
        n306 = Search and Replace String(replace all?=TRUE ("replace all? (F)"), input string=w972, search string="VgVd", replace string=w984) -> (result string=w968:string)  [unwired: 4 in, 3 out]
        n307 = Spreadsheet String To Array(format string=w970, spreadsheet string=w968, array type (2D Dbl)=w966) -> (array=w967:string[])  [unwired: 1 in]
        n308 = call "4155C Write array to file.vi"("Byte Stream File Refnum"=w975, "Header"=w967, "Data Array"=w990, "error in (no error)"=w976) -> ("dup refnum"=w973:refnum<file>, "error out"=w974:errorcluster)  [unwired: 1 in]
        n309 = Close File(refnum=w973, error in=w974) -> (error out=w962:errorcluster)  [unwired: 1 out]
      }
    }
    n310 = local write "Lines left to run:"(w39) -> ()
    n311 = Empty String/Path?(string/path=w39) -> (empty?=w75:bool)
    n312 = Not(x=w75) -> (.not. x?=w74:bool)
  }
